vi "resetCycleCounter.vi"(8 "error in (no error)":errorcluster, 11 "PreconditioningMonitor in":refnum<class "PreconditioningMonitor.lvclass">) -> (0 "error out":errorcluster, 3 "PreconditioningMonitor out":refnum<class "PreconditioningMonitor.lvclass">)   [LabVIEW 2015, in "PreconditioningMonitor.lvclass"]
uses:
  PreconditioningMonitor.lvclass
  PreconditioningMonitor.lvclass/PreconditioningMonitor.ctl
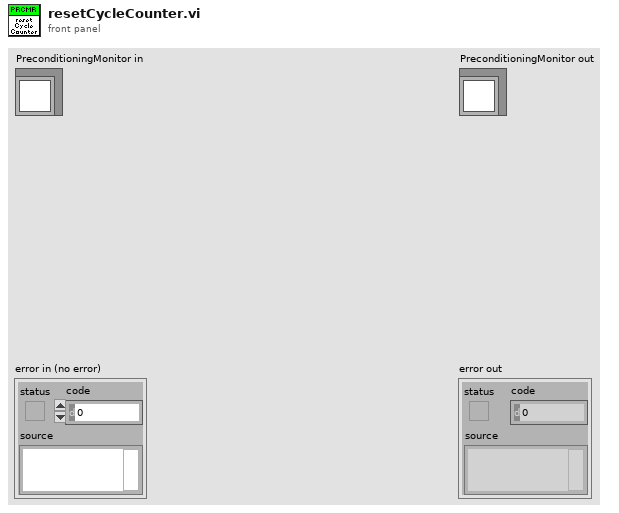
[diagram p1: front panel]
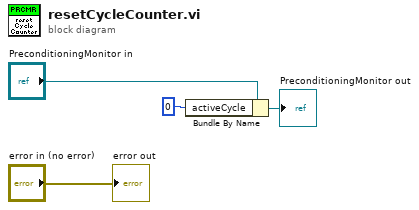
[diagram p0: block diagram]
diagram:
  n1 = Bundle By Name(cluster="PreconditioningMonitor in", "activeCycle"=u32 0) -> (→"PreconditioningMonitor out":refnum<class "PreconditioningMonitor.lvclass">)
  "error out" <- "error in (no error)"
